vi "tank.vi"() -> ()   [LabVIEW 2017]
panel:
  out "amount_out":dbl
  in  "flow_out":dbl
  in  "flow_in":dbl
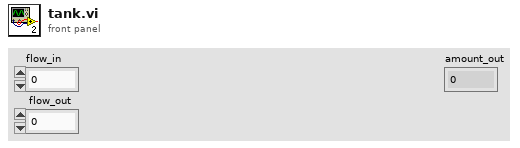
[diagram p1: front panel]
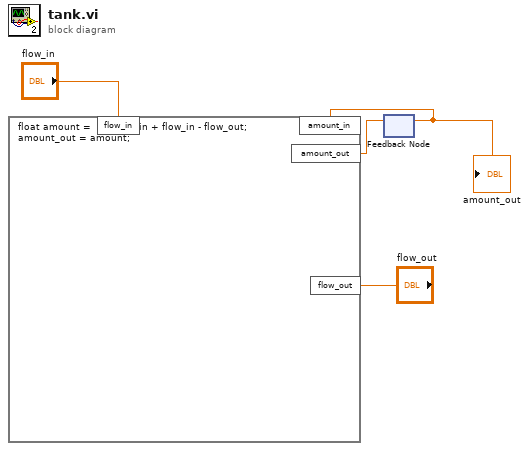
[diagram p0: block diagram]
diagram:
  n1 = feedback #1() -> (w3:dbl)  [unwired: 1 in]
  "amount_out" <- w3
  n2 = formula code="float amount =  amount_in + flow_in - flow_out;\namount_out = amount;"("flow_in"="flow_in", "amount_in"=w3, "flow_out"="flow_out") -> ("amount_out"=w4:dbl)
  n3 = feedback-in #1(w4) -> ()
